vi "Read MsgString.vi"(8 "error in (no error)":errorcluster, 11 "RealWorkActor in":refnum<class "RealWorkActor.lvclass">) -> (0 "error out":errorcluster, 2 "MsgString":string, 3 "RealWorkActor out":refnum<class "RealWorkActor.lvclass">)   [LabVIEW 2021, in "RealWorkActor.lvclass"]
uses:
  RealWorkActor.lvclass
  RealWorkActor.lvclass/RealWorkActor.ctl
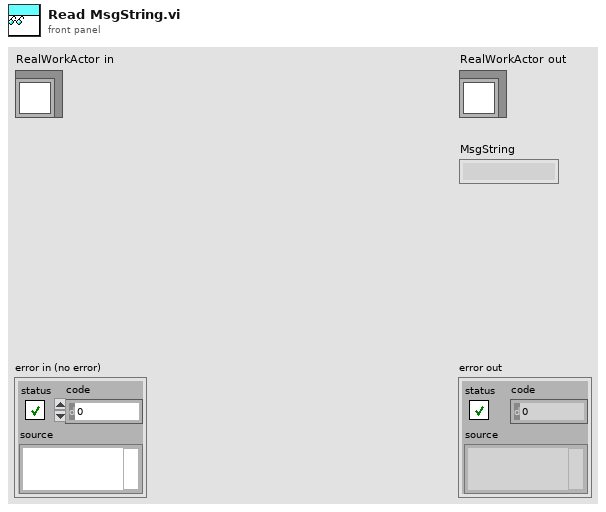
[diagram p1: front panel]
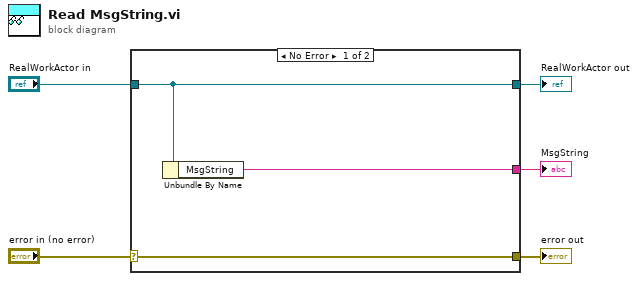
[diagram p0: block diagram]
diagram:
  n1 = case shown="No Error" "error in (no error)" {
    selector: "error in (no error)" -> [w8 w9]
    tunnel: [w8 w9] -> w4
    tunnel: [w7 w10] -> w2
    tunnel: "RealWorkActor in" -> [w7 w10]
    tunnel: [w6 _] -> w1
    frame No Error {
      n2 = Unbundle By Name(w7) -> ("MsgString"=w6:string)
    }
    frame Error {
    }
  }
  "error out" <- w4
  "RealWorkActor out" <- w2
  "MsgString" <- w1
